vi "Create subscription.vi"(8 "error in (no error)":errorcluster, 10 "Subscription ID":u64, 11 "HandleSubscribed JSON in":refnum<class "HandleSubscribed JSON.lvclass">) -> (0 "error out":errorcluster, 2 "SubscriptionDetailsParent":refnum<class "SubscriptionDetailsParent.lvclass">, 3 "HandleSubscribed JSON out":refnum<class "HandleSubscribed JSON.lvclass">)   [LabVIEW 2020, in "wamplv.lvlib" / "HandleSubscribed JSON.lvclass"]
uses:
  HandleSubscribed JSON.lvclass
  HandleSubscribed JSON.lvclass/HandleSubscribed JSON.ctl
  Message loop classes/Subscription details/SubscriptionDetails JSON/SubscriptionDetails JSON.lvclass
  C:/local/wamplv/Private/Message loop classes/Subscription details/SubscriptionDetailsParent/SubscriptionDetailsParent.lvclass
  C:/local/wamplv/Private/Requests/IContainersNotiferOrEvents/IContainersNotiferOrEvents.lvclass
  C:/local/wamplv/Private/Message loop classes/Subscription details/SubscriptionDetails JSON/SubscriptionDetails JSON.lvclass
  Message loop classes/Subscription details/SubscriptionDetailsParent/SubscriptionDetailsParent.lvclass
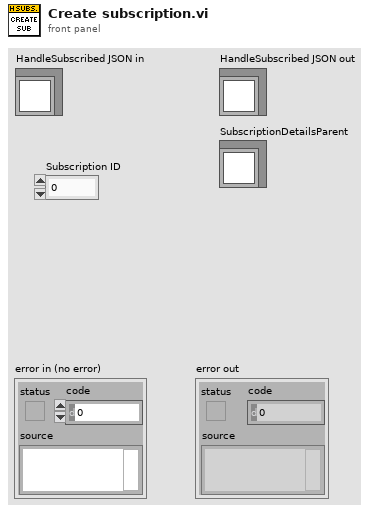
[diagram p1: front panel]
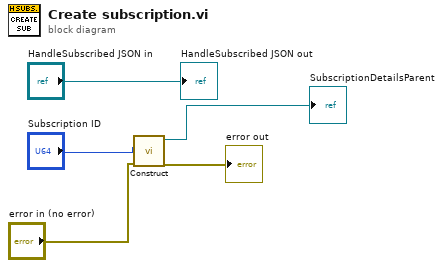
[diagram p0: block diagram]
diagram:
  n1 = call-dynamic "Construct.vi"("error in (no error)"="error in (no error)", "Subscription ID"="Subscription ID") -> ("error out"=→"error out":errorcluster, "SubscriptionDetails JSON out"=→"SubscriptionDetailsParent":refnum<class "SubscriptionDetails JSON.lvclass">)  [unwired: 8 in]
  "HandleSubscribed JSON out" <- "HandleSubscribed JSON in"
